vi "RT Error Handler - Watchdog.vi"(8 "error in (no error)":errorcluster, 11 "Message Queue":refnum<queue>) -> (3 "dup Message Queue":refnum<queue>)   [LabVIEW 2012]
uses:
  support/Message Queue/Message Cluster.ctl
  support/Message Queue/Message Queue.lvlib
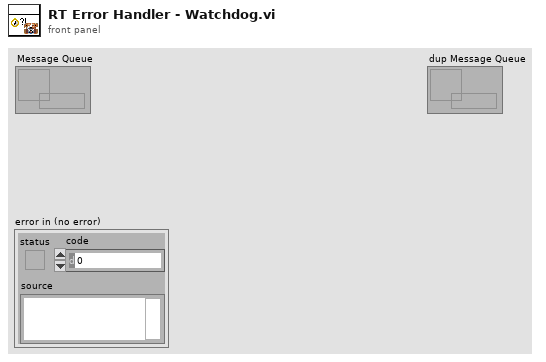
[diagram p1: front panel]
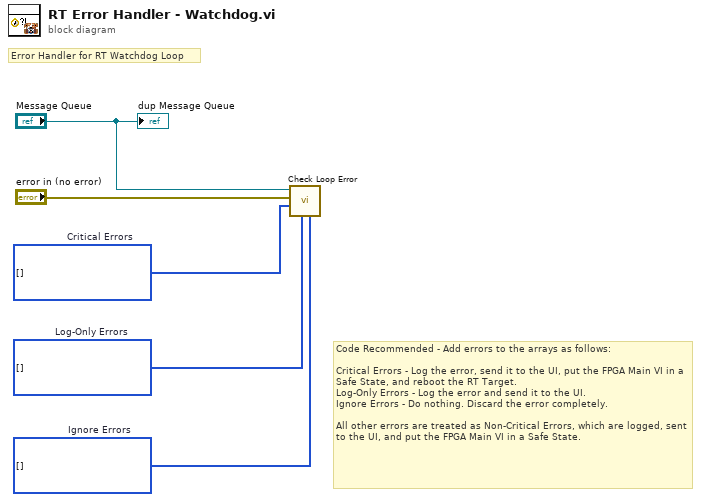
[diagram p0: block diagram]
diagram:
  w3 = i32[] []  # Ignore Errors
  w4 = i32[] []  # Log-Only Errors
  w5 = i32[] []  # Critical Errors
  # "Code Recommended - Add errors to the arrays as follows:\n\nCritical Errors - Log the error, send it to the UI, put the FPGA Main VI in a Safe State, and reboot the RT Target.\nLog-Only Errors - Log the error and send it to the UI.\nIgnore Errors - Do nothing. Discard the error completely.\n\nAll other errors are treated as Non-Critical Errors, which are logged, sent to the UI, and put the FPGA Main VI in a Safe State."
  # "Error Handler for RT Watchdog Loop"
  n1 = call "Check Loop Error.vi"("Ignore Errors"=w3, "Log-Only Errors"=w4, "Critical Errors"=w5, "error to process"="error in (no error)", "Message Queue"="Message Queue") -> ()  [unwired: 5 in, 2 out]
  "dup Message Queue" <- "Message Queue"
